vi "insert_node.vi"(7 "tree":refnum<vi>, 10 "value":i32, 11 "node":string="L 22") -> ()   [LabVIEW 2021]
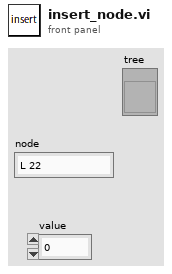
[diagram p1: front panel]
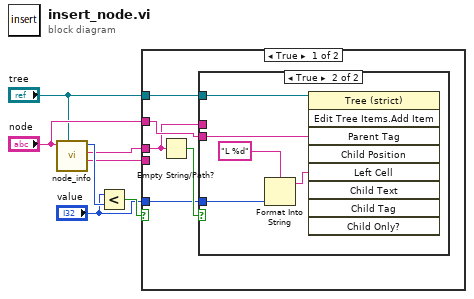
[diagram p0: block diagram]
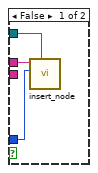
[diagram p2: hidden frame]
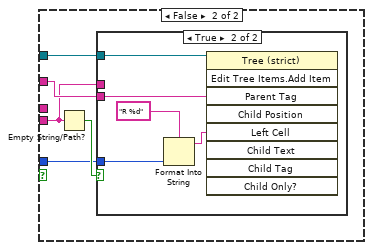
[diagram p3: hidden frame]
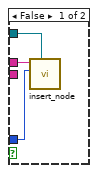
[diagram p4: hidden frame]
diagram:
  n1 = call "node_info.vi"("reference"="tree", "node"="node") -> ("right"=w2:string, "left"=w5:string, "value"=w7:i32)  [unwired: 6 in, 1 out]
  n2 = Less?(x="value", y=w7) -> (x < y?=w6:bool)
  n3 = case shown="True" w6 {
    tunnel: w5 -> [w9 _]
    tunnel: "node" -> [w11 w24]
    tunnel: "value" -> [w10 w23]
    tunnel: w2 -> [_ w21]
    tunnel: "tree" -> [w8 w22]
    frame True {
      n4 = Empty String/Path?(string/path=w9) -> (empty?=w12:bool)
      n5 = case shown="True" w12 {
        tunnel: w11 -> [_ w20]
        tunnel: w10 -> [w14 w17]
        tunnel: w9 -> [w15 _]
        tunnel: w8 -> [w13 w16]
        frame False {
          n6 = call "insert_node.vi"("tree"=w13, "value"=w14, "node"=w15) -> ()  [unwired: 9 in]
        }
        frame True {
          n7 = Format Into String(format string="L %d", w17) -> (resulting string=w18:string)  [unwired: 2 in, 1 out]
          n8 = invoke on="Invoke Node" class="Tree (strict)" method="Edit Tree Items.Add Item"(reference=w16, "Parent Tag"=w20, "Left Cell"=w18) -> ()  [unwired: 6 in, 9 out]
        }
      }
    }
    frame False {
      n9 = Empty String/Path?(string/path=w21) -> (empty?=w25:bool)
      n10 = case shown="True" w25 {
        tunnel: w24 -> [_ w33]
        tunnel: w23 -> [w27 w30]
        tunnel: w21 -> [w28 _]
        tunnel: w22 -> [w26 w29]
        frame False {
          n11 = call "insert_node.vi"("tree"=w26, "value"=w27, "node"=w28) -> ()  [unwired: 9 in]
        }
        frame True {
          n12 = Format Into String(format string="R %d", w30) -> (resulting string=w31:string)  [unwired: 2 in, 1 out]
          n13 = invoke on="Invoke Node" class="Tree (strict)" method="Edit Tree Items.Add Item"(reference=w29, "Parent Tag"=w33, "Left Cell"=w31) -> ()  [unwired: 6 in, 9 out]
        }
      }
    }
  }
